vi "Clear Buffer of Asked Questions.vi"(8 "error in (no error)":errorcluster, 11 "Controller in":refnum<class "Controller.lvclass">) -> (0 "error out":errorcluster, 3 "Controller out":refnum<class "Controller.lvclass">)   [LabVIEW 2021, in "Controller.lvlib" / "Controller.lvclass"]
uses:
  Controller.lvclass
  Controller.lvclass/Controller.ctl
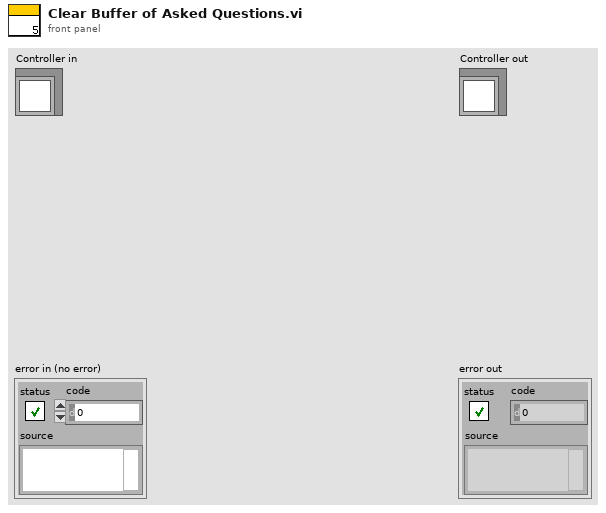
[diagram p1: front panel]
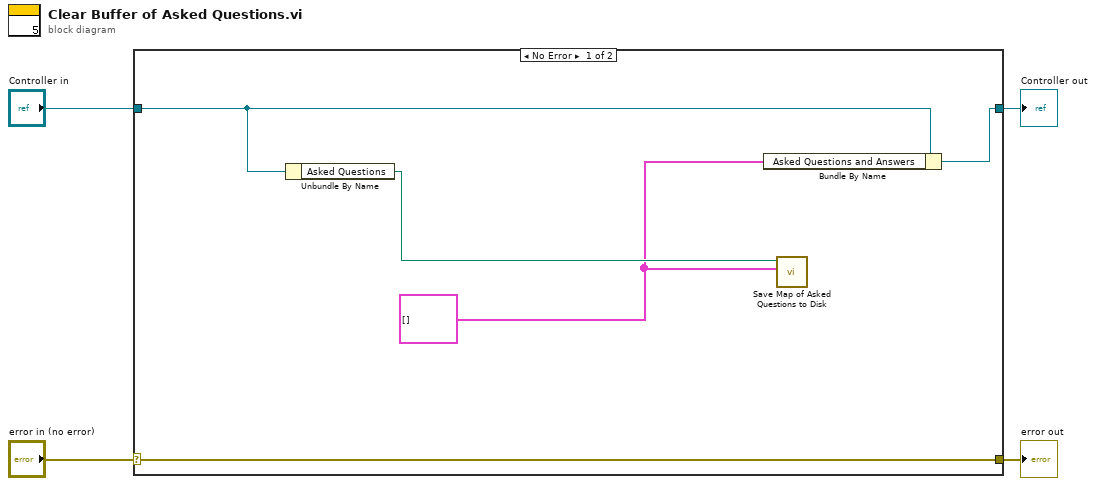
[diagram p0: block diagram]
diagram:
  n1 = case shown="No Error" "error in (no error)" {
    selector: "error in (no error)" -> [w9 w11]
    tunnel: [w9 w11] -> w3
    tunnel: [w7 w10] -> w1
    tunnel: "Controller in" -> [w8 w10]
    frame No Error {
      w5 = cluster{"String":string, "String":string}[] [] ("Asked Questions and Answers")
      n2 = Unbundle By Name(w8) -> ("Asked Questions"=w6:path)
      n3 = Bundle By Name(cluster=w8, "Asked Questions and Answers"=w5) -> (w7:refnum<class "Controller.lvclass">)
      n4 = call "Save Map of Asked Questions to Disk.vi"("Asked Questions and Answers"=w5, "Asked Questions"=w6) -> ()  [unwired: 10 in]
    }
    frame Error {
    }
  }
  "error out" <- w3
  "Controller out" <- w1
